vi "SerialsInterfaceData.vi"(1 "信息":T2, 10 "串口枚举":T3) -> (14 "串口表":map{string, refnum<class "SerialClass.lvclass">}(c390), 16 "查找结果":T1)   [LabVIEW 2019]
uses:
  02 Mode/SerialMode/SerialClass.lvclass
  <vilib>/Utility/miscctls.llb/LVMapReplaceAction.ctl
panel:
  # "所有串口连接的功能全局\n多个串口连接的存储"
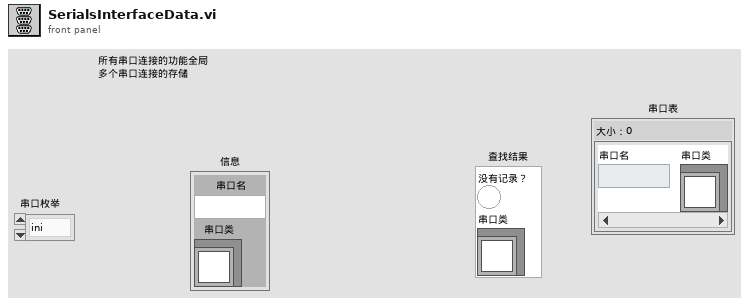
[diagram p1: front panel]
types:
  T1 = cluster{"没有记录？":bool, "串口类":refnum<class "SerialClass.lvclass">}
  T2 = cluster{"串口名":string, "串口类":refnum<class "SerialClass.lvclass">}
  T3 = typedef "串口枚举.ctl" = enum16{"ini", "增", "删", "查", "改"}
  T4 = typedef "LVMapReplaceAction.ctl" = enum32{"Modify Entry only if found", "Add or Modify Entry", "Delete Entry"}
  T5 = cluster{"key not found?":bool, "SerialClass.lvclass":refnum<class "SerialClass.lvclass">}
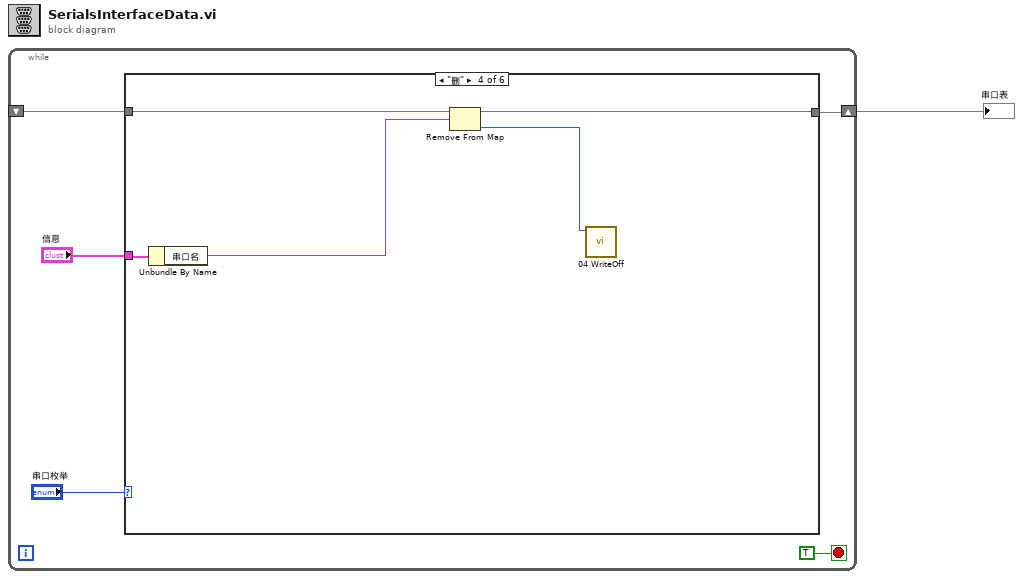
[diagram p0: block diagram]
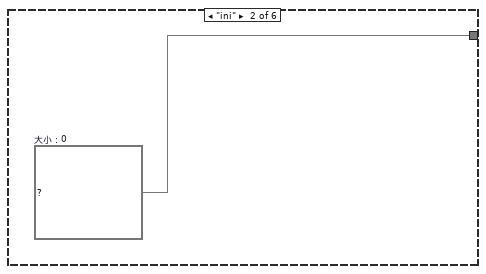
[diagram p3: hidden frame]
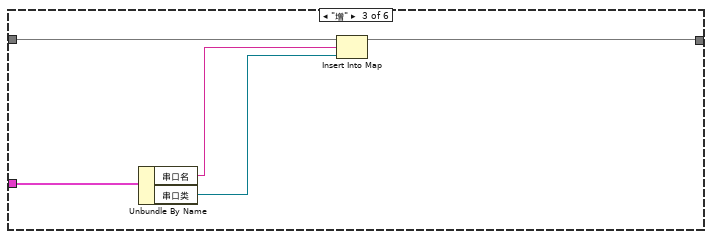
[diagram p4: hidden frame]
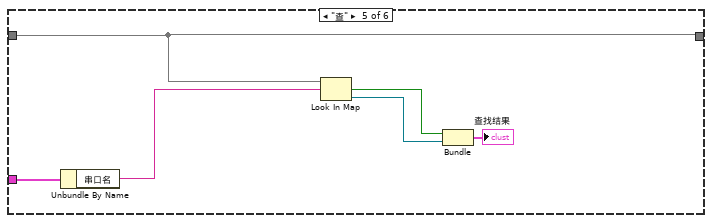
[diagram p5: hidden frame]
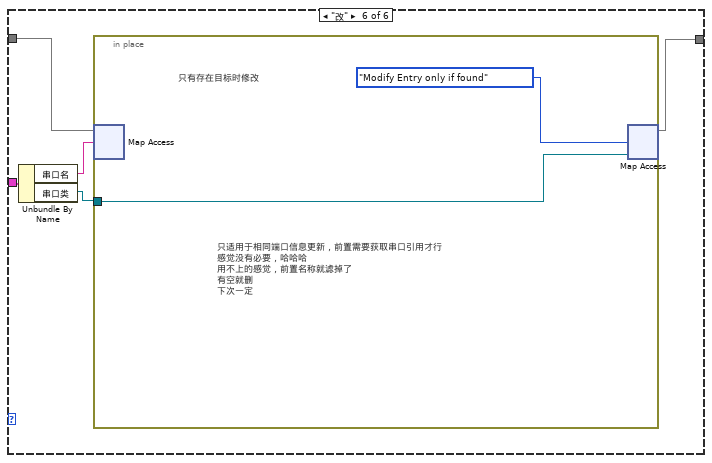
[diagram p6: hidden frame]
diagram:
  n1 = while {
    shift-right: [w4] -> w1
    shift-left: _ -> [w3]
    stop <- TRUE stop-if-true
    n2 = case shown="\"删\"" "串口枚举" {
      tunnel: [w7 w8 w12 w17 w24 w26] -> w4
      tunnel: w3 -> [w7 _ w13 w18 w24 w29]
      tunnel: "信息" -> [_ _ w9 w16 w23 w28]
      frame Default {
      }
      frame "ini" {
        w8 = map{string, refnum<class "SerialClass.lvclass">} {}  # 大小：0
      }
      frame "增" {
        n3 = Unbundle By Name(w9) -> ("串口名"=w11:string, "串口类"=w10:refnum<class "SerialClass.lvclass">)
        n4 = Insert Into Map(map in=w13, key=w11, value=w10) -> (map out=w12:map{string, refnum<class "SerialClass.lvclass">})  [unwired: 2 out]
      }
      frame "删" {
        n5 = Unbundle By Name(w16) -> ("串口名"=w15:string)
        n6 = Remove From Map(10:w15, 11:w18) -> (1:w14:refnum<class "SerialClass.lvclass">, 3:w17:map{string, refnum<class "SerialClass.lvclass">})  [unwired: 1 out]
        n7 = call-dynamic "04 WriteOff.vi"("SerialClass 输入"=w14) -> ()  [unwired: 9 in, 2 out]
      }
      frame "查" {
        n8 = Unbundle By Name(w23) -> ("串口名"=w22:string)
        n9 = Look In Map(map=w24, key=w22) -> (key not found?=w21:bool, value=w20:refnum<class "SerialClass.lvclass">)  [unwired: 1 in]
        n10 = Bundle("key not found?"=w21, "SerialClass.lvclass"=w20) -> (→"查找结果":T5)  [unwired: 1 in]
      }
      frame "改" {
        n11 = Unbundle By Name(w28) -> ("串口名"=w27:string, "串口类"=w25:refnum<class "SerialClass.lvclass">)
        n12 = in-place {
          in-place-border: w25 -> [w30]
          # "只适用于相同端口信息更新，前置需要获取串口引用才行\n感觉没有必要，哈哈哈\n用不上的感觉，前置名称就滤掉了\n有空就删\n下次一定"
          # "只有存在目标时修改"
          n13 = in-place-map #1(w29, w27) -> ()  [unwired: 1 in, 2 out]
          n14 = in-place-map #1(w30, LVMapReplaceAction."Modify Entry only if found" ("操作")) -> (w26:map{string, refnum<class "SerialClass.lvclass">})  [unwired: 2 out]
        }
      }
    }
  }
  "串口表" <- w1
